vi "Tx Packet Page.vi"(8 "error in (no error)":errorcluster, 11 "Node Ptr":T1 format="%.0x") -> (0 "error out":errorcluster)   [LabVIEW 2016, in "UDP-Custom-Device System Explorer.lvlib"]
uses:
  UDP-Custom-Device System Explorer.lvlib
  <vilib>/NI Veristand/Custom Device API/Custom Device Item Ref.ctl
  Types/TypeDef - Tx Packets Page References.ctl
  Shared/Constants.vi
  <vilib>/NI Veristand/Custom Device API/Set Item Property (I32).vi
  <vilib>/NI Veristand/Custom Device API/Set Item Property (String).vi
  <vilib>/NI Veristand/Custom Device API/Set Item Property (Boolean).vi
  <vilib>/NI Veristand/Custom Device API/Set Item Property (U16).vi
  <vilib>/NI Veristand/Custom Device API/Get Item Property (U32).vi
  <vilib>/NI Veristand/Custom Device API/Set Item Property (U32).vi
  <vilib>/NI Veristand/Custom Device API/Set Item Property (String Array).vi
  <vilib>/NI VeriStand/Custom Device API/Custom Device API.lvlib
  Shared/UDP-Custom-Device Shared.lvlib
panel:
  in  "Configure Header":bool
  in  "Endianness":u16(ring) items=["big-endian"=0, "little-endian"=2]
  in  "Auto-Assign Local NIC":bool
  in  "Port":u16
  in  "IP Address of Local NIC":string
  in  "Decimation":u16
  in  "General Header 3":cluster{"Section Name":string}={"Section Name"="Network Settings"}
  out "Packet ID":i32
  in  "Destination Port":u16
  in  "IP Address of Destination":string
  in  "Description":string
  in  "Name":string
  in  "General Header 2":cluster{"Section Name":string}={"Section Name"="Configured Channels"}
  in  "Tx Channels":i32[](listbox)
  in  "SHDocVw.IWebBrowser":refnum<k7>(container)
  in  "General Header":cluster{"Section Name":string}={"Section Name"="Packet Configuration"}
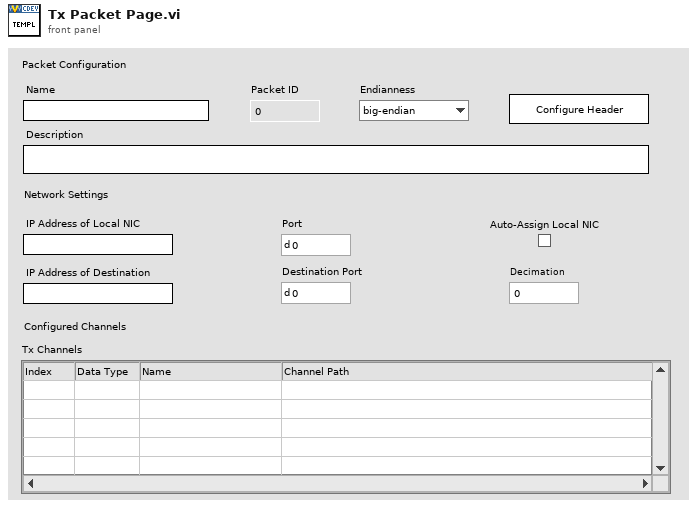
[diagram p1: front panel]
types:
  T1 = typedef "Custom Device API.lvlib/Custom Device Item Ref.ctl" = u64
  T2 = typedef "UDP-Custom-Device System Explorer.lvlib/TypeDef - Tx Packets Page References.ctl" = cluster{"Tx Channels":refnum<vi>, "Name":refnum<vi>, "Description":refnum<vi>, "Packet ID":refnum<vi>, "Dest IP Address":refnum<vi>, "Dest Port":refnum<vi>, "Decimation":refnum<vi>, "Source IP Address":refnum<vi>, "Source Port":refnum<vi>, "Auto Assign Local NIC":refnum<vi>}
  T3 = enum8{"Enabled", "Disabled", "Disabled and Grayed Out"}
  T4 = typedef "Custom Device API.lvlib/Custom Device Commands.ctl" = enum16{"Default", "Item renamed", "Shutdown", "Dynamic button pressed"}
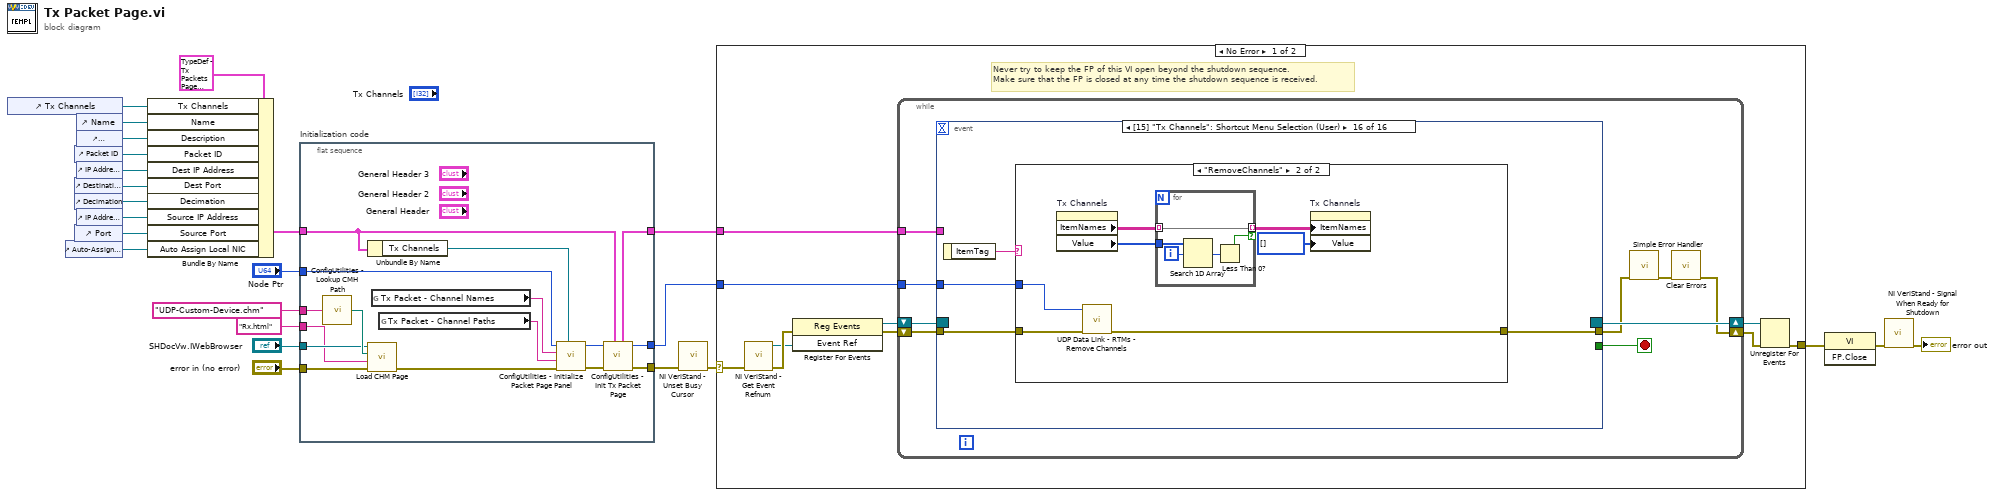
[diagram p0: block diagram]
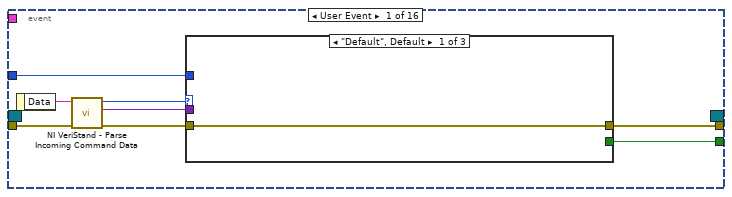
[diagram p2: hidden frame]
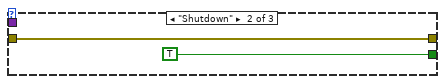
[diagram p3: hidden frame]
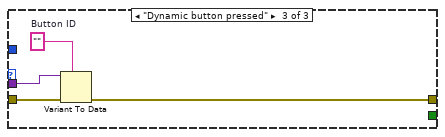
[diagram p4: hidden frame]
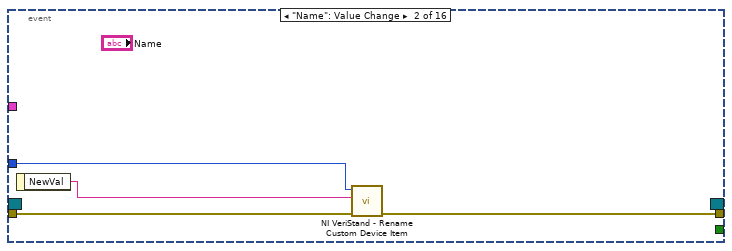
[diagram p5: hidden frame]
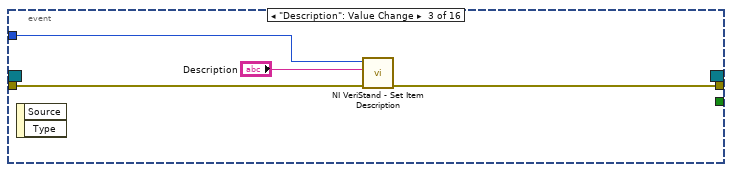
[diagram p6: hidden frame]
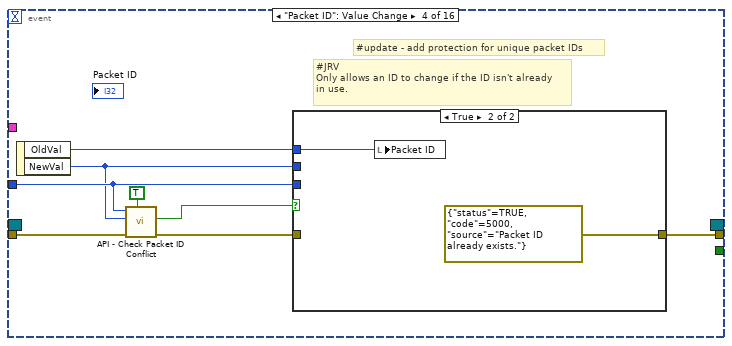
[diagram p7: hidden frame]
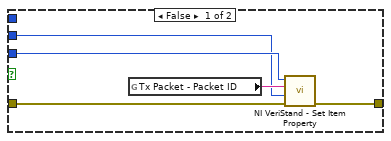
[diagram p8: hidden frame]
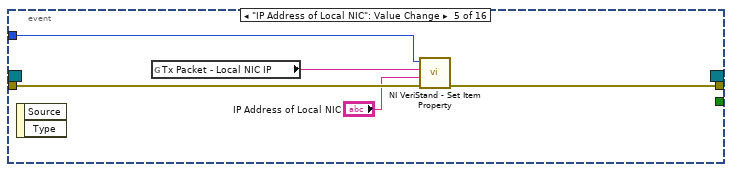
[diagram p9: hidden frame]
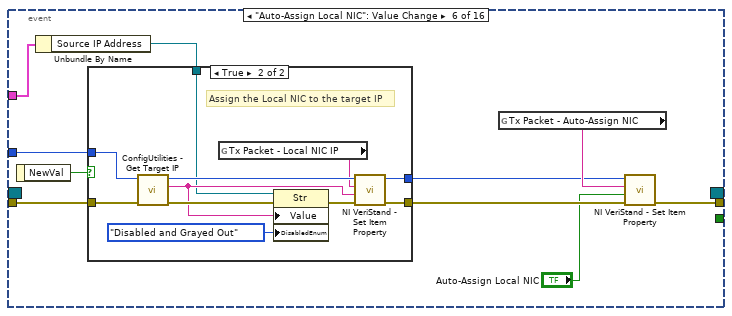
[diagram p10: hidden frame]
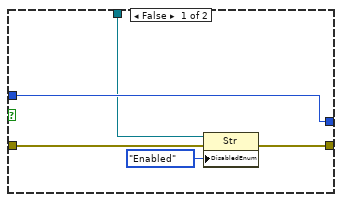
[diagram p11: hidden frame]
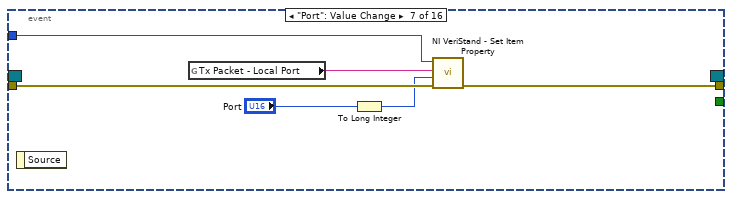
[diagram p12: hidden frame]
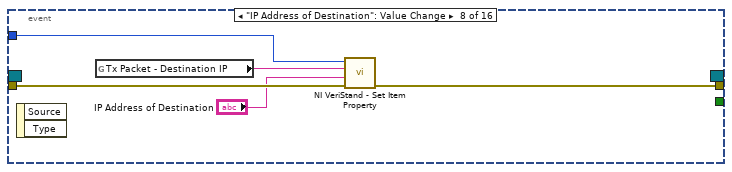
[diagram p13: hidden frame]
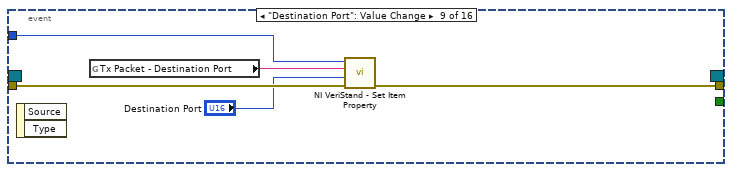
[diagram p14: hidden frame]
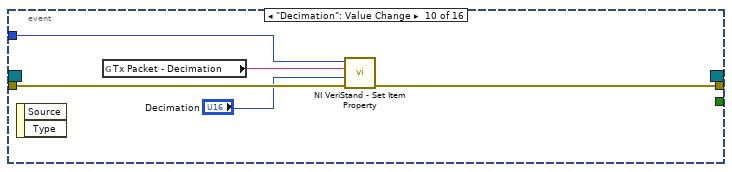
[diagram p15: hidden frame]
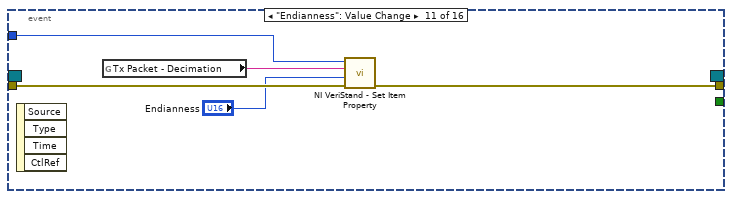
[diagram p16: hidden frame]
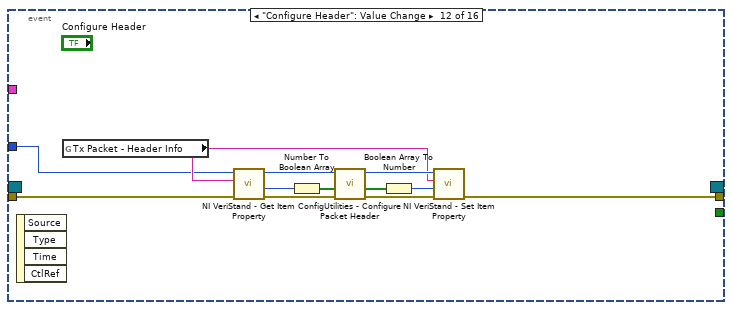
[diagram p17: hidden frame]
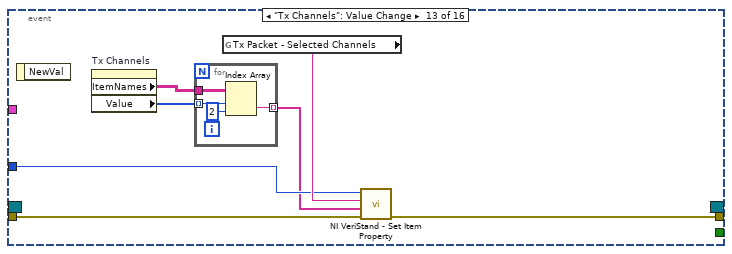
[diagram p18: hidden frame]
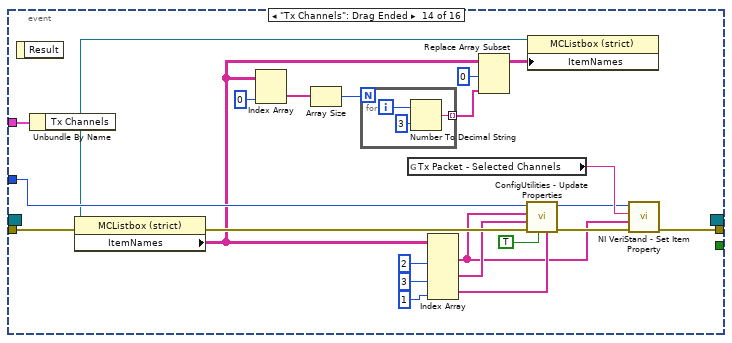
[diagram p19: hidden frame]
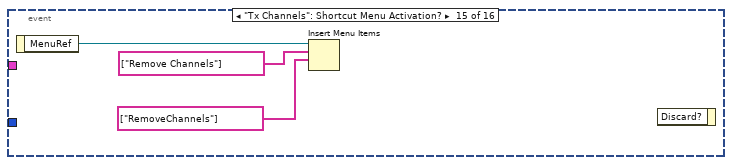
[diagram p20: hidden frame]
diagram:
  n1 = control-ref of="Tx Channels"() -> (w9:refnum<vi>)
  n2 = control-ref of="Auto-Assign Local NIC"() -> (w2:refnum<vi>)
  n3 = control-ref of="Packet ID"() -> (w5:refnum<vi>)
  n4 = control-ref of="Destination Port"() -> (w6:refnum<vi>)
  n5 = control-ref of="Decimation"() -> (w10:refnum<vi>)
  n6 = control-ref of="Port"() -> (w3:refnum<vi>)
  n7 = control-ref of="Name"() -> (w1:refnum<vi>)
  n8 = control-ref of="Description"() -> (w8:refnum<vi>)
  n9 = control-ref of="IP Address of Destination"() -> (w7:refnum<vi>)
  n10 = control-ref of="IP Address of Local NIC"() -> (w4:refnum<vi>)
  n11 = Bundle By Name(cluster=T2 {"Tx Channels"=refnum, "Name"=refnum, "Description"=refnum, "Packet ID"=refnum, "Dest IP Address"=refnum, "Dest Port"=refnum, "Decimation"=refnum, "Source IP Address"=refnum, "Source Port"=refnum, "Auto Assign Local NIC"=refnum} ("Tx Channels Section Cluster"), "Tx Channels"=w9, "Name"=w1, "Description"=w8, "Packet ID"=w5, "Dest IP Address"=w7, "Dest Port"=w6, "Decimation"=w10, "Source IP Address"=w4, "Source Port"=w3, "Auto Assign Local NIC"=w2) -> (w13:T2)
  n12 = flat-sequence "Initialization code" {
    tunnel: "error in (no error)" -> [w29]
    tunnel: "Node Ptr" -> [w40]
    tunnel: [w33] -> w20
    tunnel: [w34] -> w17
    tunnel: "SHDocVw.IWebBrowser" -> [w28]
    tunnel: "Rx.html" ("CD_CHM_Section") -> [w26]
    tunnel: "UDP-Custom-Device.chm" ("CD_CHM_FileName") -> [w27]
    tunnel: w13 -> [w32]
    tunnel: [w31] -> w12
    frame #0 {
      n13 = call "ConfigUtilities - Lookup CMH Path.vi"("Main CMH File"=w27) -> ("Compiled CMH Path"=w30:path)
      n14 = Unbundle By Name(w32) -> ("Tx Channels"=w39:refnum<vi>)
      n15 = call <vilib>:"Load CHM Page.vi"("error in (no error)"=w29, "HTML File"=w26, "Compiled CHM Path"=w30, "Web Browser Reference"=w28) -> ("error out"=w25:errorcluster)  [unwired: 7 in]
      n16 = global read "Constants.vi" "Tx Packet - Channel Names"() -> (w37:string)
      n17 = global read "Constants.vi" "Tx Packet - Channel Paths"() -> (w38:string)
      n18 = call "ConfigUtilities - Initialize Packet Page Panel.vi"("Channels Listbox"=w39, "error in (no error)"=w25, "Channel Paths Property"=w38, "Channel Names Property"=w37, "Item Ref in"=w40) -> ("error out"=w36:errorcluster, "Item Ref out"=w35:T1)  [unwired: 3 in, 2 out]
      n19 = call "ConfigUtilities - Init Tx Packet Page.vi"("Tx Packets Cluster In"=w32, "error in (no error)"=w36, "Node Ptr In"=w35) -> ("error out"=w33:errorcluster, "Node Ptr Out"=w34:T1, "Tx Packets Cluster Out"=w31:T2)  [unwired: 6 in]
    }
  }
  n20 = call <vilib>:"NI VeriStand - Unset Busy Cursor.vi"("error in (no error)"=w20) -> ("error out"=w19:errorcluster)  [unwired: 10 out]
  n21 = case shown="No Error" w19 {
    selector: w19 -> [w42 w226]
    tunnel: [w47 w224] -> w24
    tunnel: w17 -> [w43 _]
    tunnel: w12 -> [w41 _]
    frame No Error {
      # "Never try to keep the FP of this VI open beyond the shutdown sequence.\nMake sure that the FP is closed at any time the shutdown sequence is received."
      n22 = call <vilib>:"NI VeriStand - Get Event Refnum.vi"("error in (no error)"=w42) -> ("error out"=w50:errorcluster, "Event Ref"=w46:refnum<user-event>)  [unwired: 9 out]
      n23 = register-events(error in=w50, w46) -> (reference out=w44:refnum<event-registration>, error out=w45:errorcluster)  [unwired: 1 in]
      n24 = while {
        tunnel: w43 -> [w55]
        shift-right: [w52] -> w48
        shift-left: w45 -> [w58]
        shift-right: [w59] -> w49
        shift-left: w44 -> [w57]
        tunnel: w41 -> [w51]
        stop <- w56 stop-if-true
        n25 = event shown="[15] \"Tx Channels\": Shortcut Menu Selection (User)" {
          selector: w57 -> [_ _ _ _ _ _ _ _ _ _ _ _ _ _ _ _]
          dyn-events: [_ _ _ _ _ _ _ _ _ _ _ _ _ _ _ _] -> w59
          timeout: _ -> [_ _ _ _ _ _ _ _ _ _ _ _ _ _ _ _]
          tunnel: w58 -> [w67 w78 w82 w84 w101 w111 w133 w139 w144 w149 w154 w157 w169 w200 _ w208]
          tunnel: [w63 _ _ _ _ _ _ _ _ _ _ _ _ _ _ _] -> w56
          tunnel: [w62 w76 w79 w90 w98 w110 w130 w136 w141 w146 w151 w156 w167 w197 _ w207] -> w54
          tunnel: w55 -> [w61 w77 w81 w87 w99 w107 w132 w137 w142 w147 w152 w155 w170 w194 _ w209]
          tunnel: w51 -> [_ _ _ _ _ w106 _ _ _ _ _ _ _ w192 _ _]
          event User Event {
            n26 = event-data() -> ("Data"=w66:string)  [unwired: 1 out]
            n27 = call <vilib>:"NI VeriStand - Parse Incoming Command Data.vi"("error in (no error)"=w67, "Incoming data"=w66) -> ("error out"=w65:errorcluster, "Outgoing data"=w60:variant, "Action"=w64:T4)  [unwired: 7 out]
            n28 = case shown="\"Default\", Default" w64 {
              tunnel: w65 -> [w68 w69 w74]
              tunnel: [_ TRUE _] -> w63
              tunnel: [w68 w69 w71] -> w62
              tunnel: w61 -> [_ _ _]
              tunnel: w60 -> [_ _ w73]
              frame "Default", Default {
              }
              frame "Shutdown" {
              }
              frame "Dynamic button pressed" {
                w72 = ""  # Button ID
                n29 = Variant To Data(error in=w74, type=w72, Variant=w73) -> (error out=w71:errorcluster)  [unwired: 1 out]
              }
            }
          }
          event "Name": Value Change {
            n30 = event-data() -> ("NewVal"=w75:string)  [unwired: 1 out]
            n31 = call <vilib>:"NI VeriStand - Rename Custom Device Item.vi"("error in (no error)"=w78, "New Name"=w75, "Item Ref in"=w77) -> ("error out"=w76:errorcluster)  [unwired: 6 in, 2 out]
          }
          event "Description": Value Change {
            n32 = event-data() -> ()  [unwired: 3 out]
            n33 = call <vilib>:"NI VeriStand - Set Item Description.vi"("error in (no error)"=w82, "Description"="Description", "Item Ref in"=w81) -> ("error out"=w79:errorcluster)  [unwired: 6 in, 2 out]
          }
          event "Packet ID": Value Change {
            # "#JRV\nOnly allows an ID to change if the ID isn't already\nin use."
            # "#update - add protection for unique packet IDs"
            n34 = event-data() -> ("OldVal"=w89:i32, "NewVal"=w86:i32)  [unwired: 1 out]
            n35 = call "API - Check Packet ID Conflict.vi"("Transmit?"=TRUE, "error in (no error)"=w84, "New ID"=w86, "Packet Ref In"=w87) -> ("error out"=w83:errorcluster, "Conflicting ID?"=w85:bool)  [unwired: 6 in]
            n36 = case shown="True" w85 {
              tunnel: w83 -> [w95 _]
              tunnel: w87 -> [w94 _]
              tunnel: [w93 errorcluster {"status"=TRUE, "code"=5000, "source"="Packet ID already exists."} ("error out")] -> w90
              tunnel: w89 -> [_ w97]
              tunnel: w86 -> [w91 _]
              frame False {
                n37 = global read "Constants.vi" "Tx Packet - Packet ID"() -> (w92:string)
                n38 = call-poly <vilib>:"NI VeriStand - Set Item Property.vi"("error in (no error)"=w95, "Value"=w91, "Property Name"=w92, "Item Ref in"=w94) -> ("error out"=w93:errorcluster)  [unwired: 5 in, 2 out]
              }
              frame True {
                n39 = local write "Packet ID"(w97) -> ()
              }
            }
          }
          event "IP Address of Local NIC": Value Change {
            n40 = event-data() -> ()  [unwired: 3 out]
            n41 = global read "Constants.vi" "Tx Packet - Local NIC IP"() -> (w102:string)
            n42 = call-poly <vilib>:"NI VeriStand - Set Item Property.vi"("error in (no error)"=w101, "Value"="IP Address of Local NIC", "Property Name"=w102, "Item Ref in"=w99) -> ("error out"=w98:errorcluster)  [unwired: 5 in, 2 out]
          }
          event "Auto-Assign Local NIC": Value Change {
            n43 = event-data() -> ("NewVal"=w105:bool)  [unwired: 1 out]
            n44 = Unbundle By Name(w106) -> ("Source IP Address"=w104:refnum<vi>)
            n45 = case shown="True" w105 {
              tunnel: w111 -> [w117 w122]
              tunnel: [w115 w121] -> w109
              tunnel: [w114 w120] -> w108
              tunnel: w107 -> [w114 w119]
              tunnel: w104 -> [w113 w118]
              frame False {
                n46 = property class="Str"(reference=w113, error in=w117, "DisabledEnum"=T3."Enabled" ("Disabled")) -> (error out=w115:errorcluster)  [unwired: 1 out]
              }
              frame True {
                # "Assign the Local NIC to the target IP"
                n47 = call "ConfigUtilities - Get Target IP.vi"("error in"=w122, "Item Ref in"=w119) -> ("error out"=w128:errorcluster, "IPAddress"=w125:string, "Item Ref out"=w127:T1)  [unwired: 7 in]
                n48 = global read "Constants.vi" "Tx Packet - Local NIC IP"() -> (w126:string)
                n49 = property class="Str"(reference=w118, error in=w128, "Value"=w125, "DisabledEnum"=T3."Disabled and Grayed Out" ("Disabled")) -> (error out=w123:errorcluster)  [unwired: 1 out]
                n50 = call-poly <vilib>:"NI VeriStand - Set Item Property.vi"("error in (no error)"=w123, "Value"=w125, "Property Name"=w126, "Item Ref in"=w127) -> ("error out"=w121:errorcluster, "Item Ref out"=w120:T1)  [unwired: 5 in, 1 out]
              }
            }
            n51 = global read "Constants.vi" "Tx Packet - Auto-Assign NIC"() -> (w112:string)
            n52 = call-poly <vilib>:"NI VeriStand - Set Item Property.vi"("error in (no error)"=w109, "Value"="Auto-Assign Local NIC", "Property Name"=w112, "Item Ref in"=w108) -> ("error out"=w110:errorcluster)  [unwired: 5 in, 2 out]
          }
          event "Port": Value Change {
            n53 = event-data() -> ()  [unwired: 2 out]
            n54 = global read "Constants.vi" "Tx Packet - Local Port"() -> (w134:string)
            n55 = To Long Integer(number="Port") -> (32bit integer=w129:i32)
            n56 = call-poly <vilib>:"NI VeriStand - Set Item Property.vi"("error in (no error)"=w133, "Value"=w129, "Property Name"=w134, "Item Ref in"=w132) -> ("error out"=w130:errorcluster)  [unwired: 5 in, 2 out]
          }
          event "IP Address of Destination": Value Change {
            n57 = event-data() -> ()  [unwired: 3 out]
            n58 = global read "Constants.vi" "Tx Packet - Destination IP"() -> (w138:string)
            n59 = call-poly <vilib>:"NI VeriStand - Set Item Property.vi"("error in (no error)"=w139, "Value"="IP Address of Destination", "Property Name"=w138, "Item Ref in"=w137) -> ("error out"=w136:errorcluster)  [unwired: 5 in, 2 out]
          }
          event "Destination Port": Value Change {
            n60 = event-data() -> ()  [unwired: 3 out]
            n61 = global read "Constants.vi" "Tx Packet - Destination Port"() -> (w143:string)
            n62 = call-poly <vilib>:"NI VeriStand - Set Item Property.vi"("error in (no error)"=w144, "Value"="Destination Port", "Property Name"=w143, "Item Ref in"=w142) -> ("error out"=w141:errorcluster)  [unwired: 5 in, 2 out]
          }
          event "Decimation": Value Change {
            n63 = event-data() -> ()  [unwired: 3 out]
            n64 = global read "Constants.vi" "Tx Packet - Decimation"() -> (w148:string)
            n65 = call-poly <vilib>:"NI VeriStand - Set Item Property.vi"("error in (no error)"=w149, "Value"="Decimation", "Property Name"=w148, "Item Ref in"=w147) -> ("error out"=w146:errorcluster)  [unwired: 5 in, 2 out]
          }
          event "Endianness": Value Change {
            n66 = event-data() -> ()  [unwired: 5 out]
            n67 = global read "Constants.vi" "Tx Packet - Decimation"() -> (w153:string)
            n68 = call-poly <vilib>:"NI VeriStand - Set Item Property.vi"("error in (no error)"=w154, "Value"="Endianness", "Property Name"=w153, "Item Ref in"=w152) -> ("error out"=w151:errorcluster)  [unwired: 5 in, 2 out]
          }
          event "Configure Header": Value Change {
            n69 = event-data() -> ()  [unwired: 5 out]
            n70 = global read "Constants.vi" "Tx Packet - Header Info"() -> (w158:string)
            n71 = call-poly <vilib>:"NI VeriStand - Get Item Property.vi"("error in (no error)"=w157, "Property Name"=w158, "Item Ref in"=w155) -> ("error out"=w166:errorcluster, "Value"=w163:u32, "Item Ref out"=w165:T1)  [unwired: 5 in, 1 out]
            n72 = Number To Boolean Array(number=w163) -> (Boolean array=w164:bool[])
            n73 = call "ConfigUtilities - Configure Packet Header.vi"("error in (no error)"=w166, "Header Elements In"=w164, "Packet Ref in"=w165) -> ("error out"=w162:errorcluster, "Header Elements Out"=w161:bool[], "Packet Ref out"=w159:T1)  [unwired: 6 in]
            n74 = Boolean Array To Number(Boolean array=w161) -> (number=w160:u32)
            n75 = call-poly <vilib>:"NI VeriStand - Set Item Property.vi"("error in (no error)"=w162, "Value"=w160, "Property Name"=w158, "Item Ref in"=w159) -> ("error out"=w156:errorcluster)  [unwired: 5 in, 2 out]
          }
          event "Tx Channels": Value Change {
            n76 = event-data() -> ()  [unwired: 2 out]
            n77 = property on="Tx Channels" class="MCListbox (strict)"() -> ("ItemNames"=w172:string[][], "Value"=w173:i32[])  [unwired: 2 in, 2 out]
            n78 = for {
              tunnel: w172 -> [w177]
              tunnel: [w176] -> w168 mode=indexing
              tunnel: w173 -> [w175] mode=indexing
              n79 = Index Array(array=w177, index (row)=w175, index (col)=2 ("disabled index (row)")) -> (element=w176:string)
            }
            n80 = global read "Constants.vi" "Tx Packet - Selected Channels"() -> (w171:string)
            n81 = call-poly <vilib>:"NI VeriStand - Set Item Property.vi"("error in (no error)"=w169, "Value"=w168, "Property Name"=w171, "Item Ref in"=w170) -> ("error out"=w167:errorcluster)  [unwired: 5 in, 2 out]
          }
          event "Tx Channels": Drag Ended {
            n82 = event-data() -> ()  [unwired: 2 out]
            n83 = Unbundle By Name(w192) -> ("Tx Channels"=w187:refnum<vi>)
            n84 = property class="MCListbox (strict)"(reference=w187, error in=w200) -> (error out=w199:errorcluster, "ItemNames"=w184:string[][])  [unwired: 1 out]
            n85 = Index Array(array=w184, index (col)=0 ("disabled index (col)")) -> (element=w186:string[])  [unwired: 1 in]
            n86 = Array Size(array=w186) -> (size(s)=w185:i32)
            n87 = for {
              N: w185 -> [_]
              tunnel: [w201] -> w182 mode=indexing
              i -> [w203]
              n88 = Number To Decimal String(number=w203, width (-)=i16 3) -> (decimal integer string=w201:string)
            }
            n89 = global read "Constants.vi" "Tx Packet - Selected Channels"() -> (w196:string)
            n90 = Index Array(array=w184, index (col) #1=2 ("index (row)"), index (col) #2=3 ("index (col)"), index (col) #3=1 ("index (col)")) -> (element #1=w178:string[], element #2=w193:string[], element #3=w179:string[])  [unwired: 3 in]
            n91 = Replace Array Subset(array=w184, new element=w182, index (col)=0 ("disabled index (col)")) -> (w181:string[][])  [unwired: 1 in]
            n92 = call "ConfigUtilities - Update Properties.vi"("Channel Data Types"=w179, "Tx?"=TRUE, "error in (no error)"=w199, "Channel Paths"=w193, "Channel Names"=w178, "Item Ref in"=w194) -> ("error out"=w198:errorcluster, "Item Ref out"=w195:T1)  [unwired: 4 in]
            n93 = property class="MCListbox (strict)"(reference=w187, "ItemNames"=w181) -> ()  [unwired: 1 in, 2 out]
            n94 = call-poly <vilib>:"NI VeriStand - Set Item Property.vi"("error in (no error)"=w198, "Value"=w178, "Property Name"=w196, "Item Ref in"=w195) -> ("error out"=w197:errorcluster)  [unwired: 5 in, 2 out]
          }
          event "Tx Channels": Shortcut Menu Activation? {
            n95 = event-data() -> ("MenuRef"=w204:refnum<k9>)  [unwired: 1 out]
            n96 = Insert Menu Items(7:string[] ["RemoveChannels"] ("item names"), 8:string[] ["Remove Channels"] ("item names"), 9:w204) -> ()  [unwired: 3 in, 3 out]
            n97 = event-data() -> ()  [unwired: 2 in, 1 out]
          }
          event "Tx Channels": Shortcut Menu Selection (User) {
            n98 = event-data() -> ("ItemTag"=w210:string)  [unwired: 1 out]
            n99 = case shown="\"RemoveChannels\"" w210 {
              tunnel: w209 -> [_ w218]
              tunnel: w208 -> [w211 w217]
              tunnel: [w211 w212] -> w207
              frame "False", Default {
              }
              frame "RemoveChannels" {
                n100 = property on="Tx Channels" class="MCListbox (strict)"() -> ("ItemNames"=w216:string[][], "Value"=w215:i32[])  [unwired: 2 in, 2 out]
                n101 = call "UDP Data Link - RTMs - Remove Channels.vi"("error in (no error)"=w217, "Node Ptr"=w218) -> ("error out"=w212:errorcluster)  [unwired: 9 in]
                n102 = for {
                  tunnel: w215 -> [w222]
                  tunnel: [w223] -> w214 mode=indexing if=w219
                  tunnel: w216 -> [w223] mode=indexing
                  i -> [w221]
                  n103 = Search 1D Array(1D array=w222, element=w221) -> (index of element=w220:i32)  [unwired: 1 in]
                  n104 = Less Than 0?(x=w220) -> (x < 0?=w219:bool)
                }
                n105 = property on="Tx Channels" class="MCListbox (strict)"("ItemNames"=w214, "Value"=i32[] [] ("Tx Channels")) -> ()  [unwired: 2 in, 2 out]
              }
            }
          }
        }
        n106 = call <vilib>:"Simple Error Handler.vi"("error in (no error)"=w54) -> ("error out"=w53:errorcluster)  [unwired: 1 in, 7 out]
        n107 = call <vilib>:"Clear Errors.vi"("error in (no error)"=w53) -> ("error out"=w52:errorcluster)  [unwired: 1 in, 5 out]
      }
      n108 = Unregister For Events(event registration refnum=w49, error in=w48) -> (error out=w47:errorcluster)
    }
    frame Error {
      n109 = call <vilib>:"Simple Error Handler.vi"("error in (no error)"=w226) -> ("error out"=w225:errorcluster)  [unwired: 1 in, 7 out]
      n110 = call <vilib>:"Clear Errors.vi"("error in (no error)"=w225) -> ("error out"=w224:errorcluster)  [unwired: 1 in, 5 out]
    }
  }
  n111 = invoke class="VI" method="FP.Close"(error in=w24) -> (error out=w23:errorcluster)  [unwired: 2 in, 2 out]
  n112 = call <vilib>:"NI VeriStand - Signal When Ready for Shutdown.vi"("error in (no error)"=w23) -> ("error out"=→"error out":errorcluster)  [unwired: 10 out]
